vi "TCPPacket Write Header.vi"(8 "error in (no error)":errorcluster, 11 "TCPPacket in":refnum<class "TCPPacket.lvclass">) -> (0 "error out":errorcluster, 2 "Data":u8[](array[numeric]), 3 "TCPPacket out":refnum<class "TCPPacket.lvclass">)   [LabVIEW 2019, in "TCPPacket.lvclass"]
uses:
  TCPPacket.lvclass
  TCPPacket.lvclass/TCPPacket.ctl
  <vilib>/addons/_JKI.lib/Serialization/JSON/JKI JSON Serialization.lvlib
  <vilib>/addons/Tools/Unicode/UTF8 Tools.lvlib
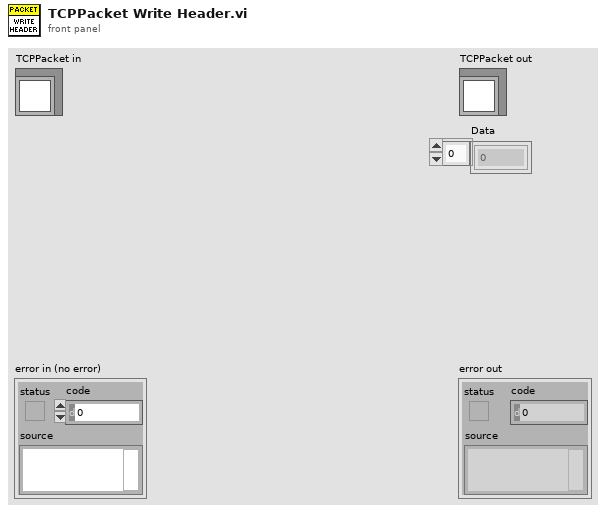
[diagram p1: front panel]
types:
  T1 = typedef "TCPPacket.lvclass/TCPHeader STYP.ctl" = cluster{"byteorder":string, "content-length":u32, "content-type":string, "content-encoding":string}
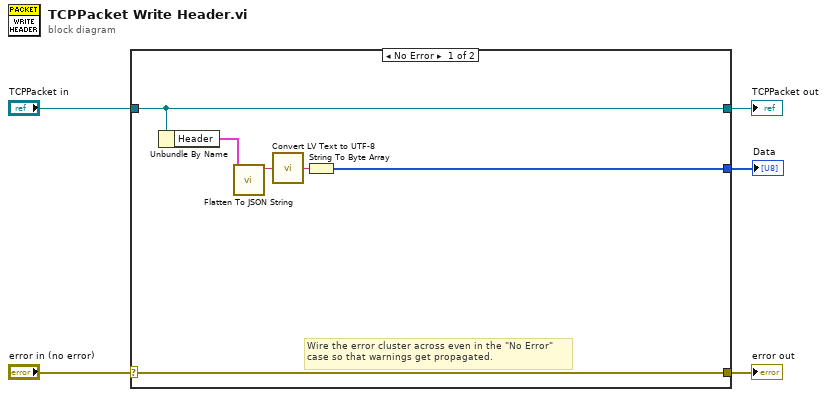
[diagram p0: block diagram]
diagram:
  n1 = case shown="No Error" "error in (no error)" {
    selector: "error in (no error)" -> [w11 w13]
    tunnel: [w11 w13] -> w4
    tunnel: [w10 w12] -> w2
    tunnel: "TCPPacket in" -> [w10 w12]
    tunnel: [w6 _] -> w1
    frame No Error {
      # "Wire the error cluster across even in the \"No Error\"\ncase so that warnings get propagated."
      n2 = Unbundle By Name(w10) -> ("Header"=w9:T1)
      n3 = call <vilib>:"Flatten To JSON String.vi"("Variant"=w9) -> ("JSON String"=w8:string)  [unwired: 9 in, 1 out]
      n4 = call <vilib>:"Convert LV Text to UTF-8.vi"("LV Text"=w8) -> ("UTF-8 Text"=w7:string)  [unwired: 13 in, 1 out]
      n5 = String To Byte Array(string=w7) -> (unsigned byte array=w6:u8[])
    }
    frame Error {
    }
  }
  "error out" <- w4
  "TCPPacket out" <- w2
  "Data" <- w1
